vi "Teleop Arm.vi"   [LabVIEW 2011]
types:
  T1 = cluster{"Buttons":cluster{"A":bool, "B":bool, "X":bool, "Y":bool, "Left Bumper":bool, "Right Bumper":bool, "Back":bool, "Start":bool, "Left Thumbstick":bool, "Right Thumbstick":bool}, "Axes":cluster{"Left X ":dbl, "Left Y":dbl, "Triggers":dbl, "Right Stick X":dbl, "Right Stick Y":dbl, "D-Pad X":dbl}}
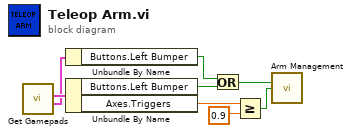
[diagram p0: block diagram]
diagram:
  n1 = call "Get Gamepads.vi"() -> ("Secondary"=w2:T1, "Driver"=w3:T1)  [unwired: 10 in]
  n2 = Unbundle By Name(w2) -> ("Buttons.Left Bumper"=w8:bool)
  n3 = Unbundle By Name(w3) -> ("Buttons.Left Bumper"=w7:bool, "Axes.Triggers"=w4:dbl)
  n4 = Or(x=w8, y=w7) -> (x .or. y?=w6:bool)
  n5 = Greater Or Equal?(x=w4, y=0.9) -> (x >= y?=w1:bool)
  n6 = call "Arm Management.vi"("Up Button"=w6, "Down Button"=w1) -> ()  [unwired: 14 in]
